vi "main.vi"(8 "error in":errorcluster caption="错误输入") -> (0 "error out":errorcluster caption="错误输出", 3 "task out":refnum<k21> caption="任务输出")   [LabVIEW 2019]
uses:
  <vilib>/DAQmx/create/channels.llb/DAQmx Create Channel (AI-Voltage-Basic).vi
  <vilib>/DAQmx/configure/timing.llb/DAQmx Timing (Sample Clock).vi
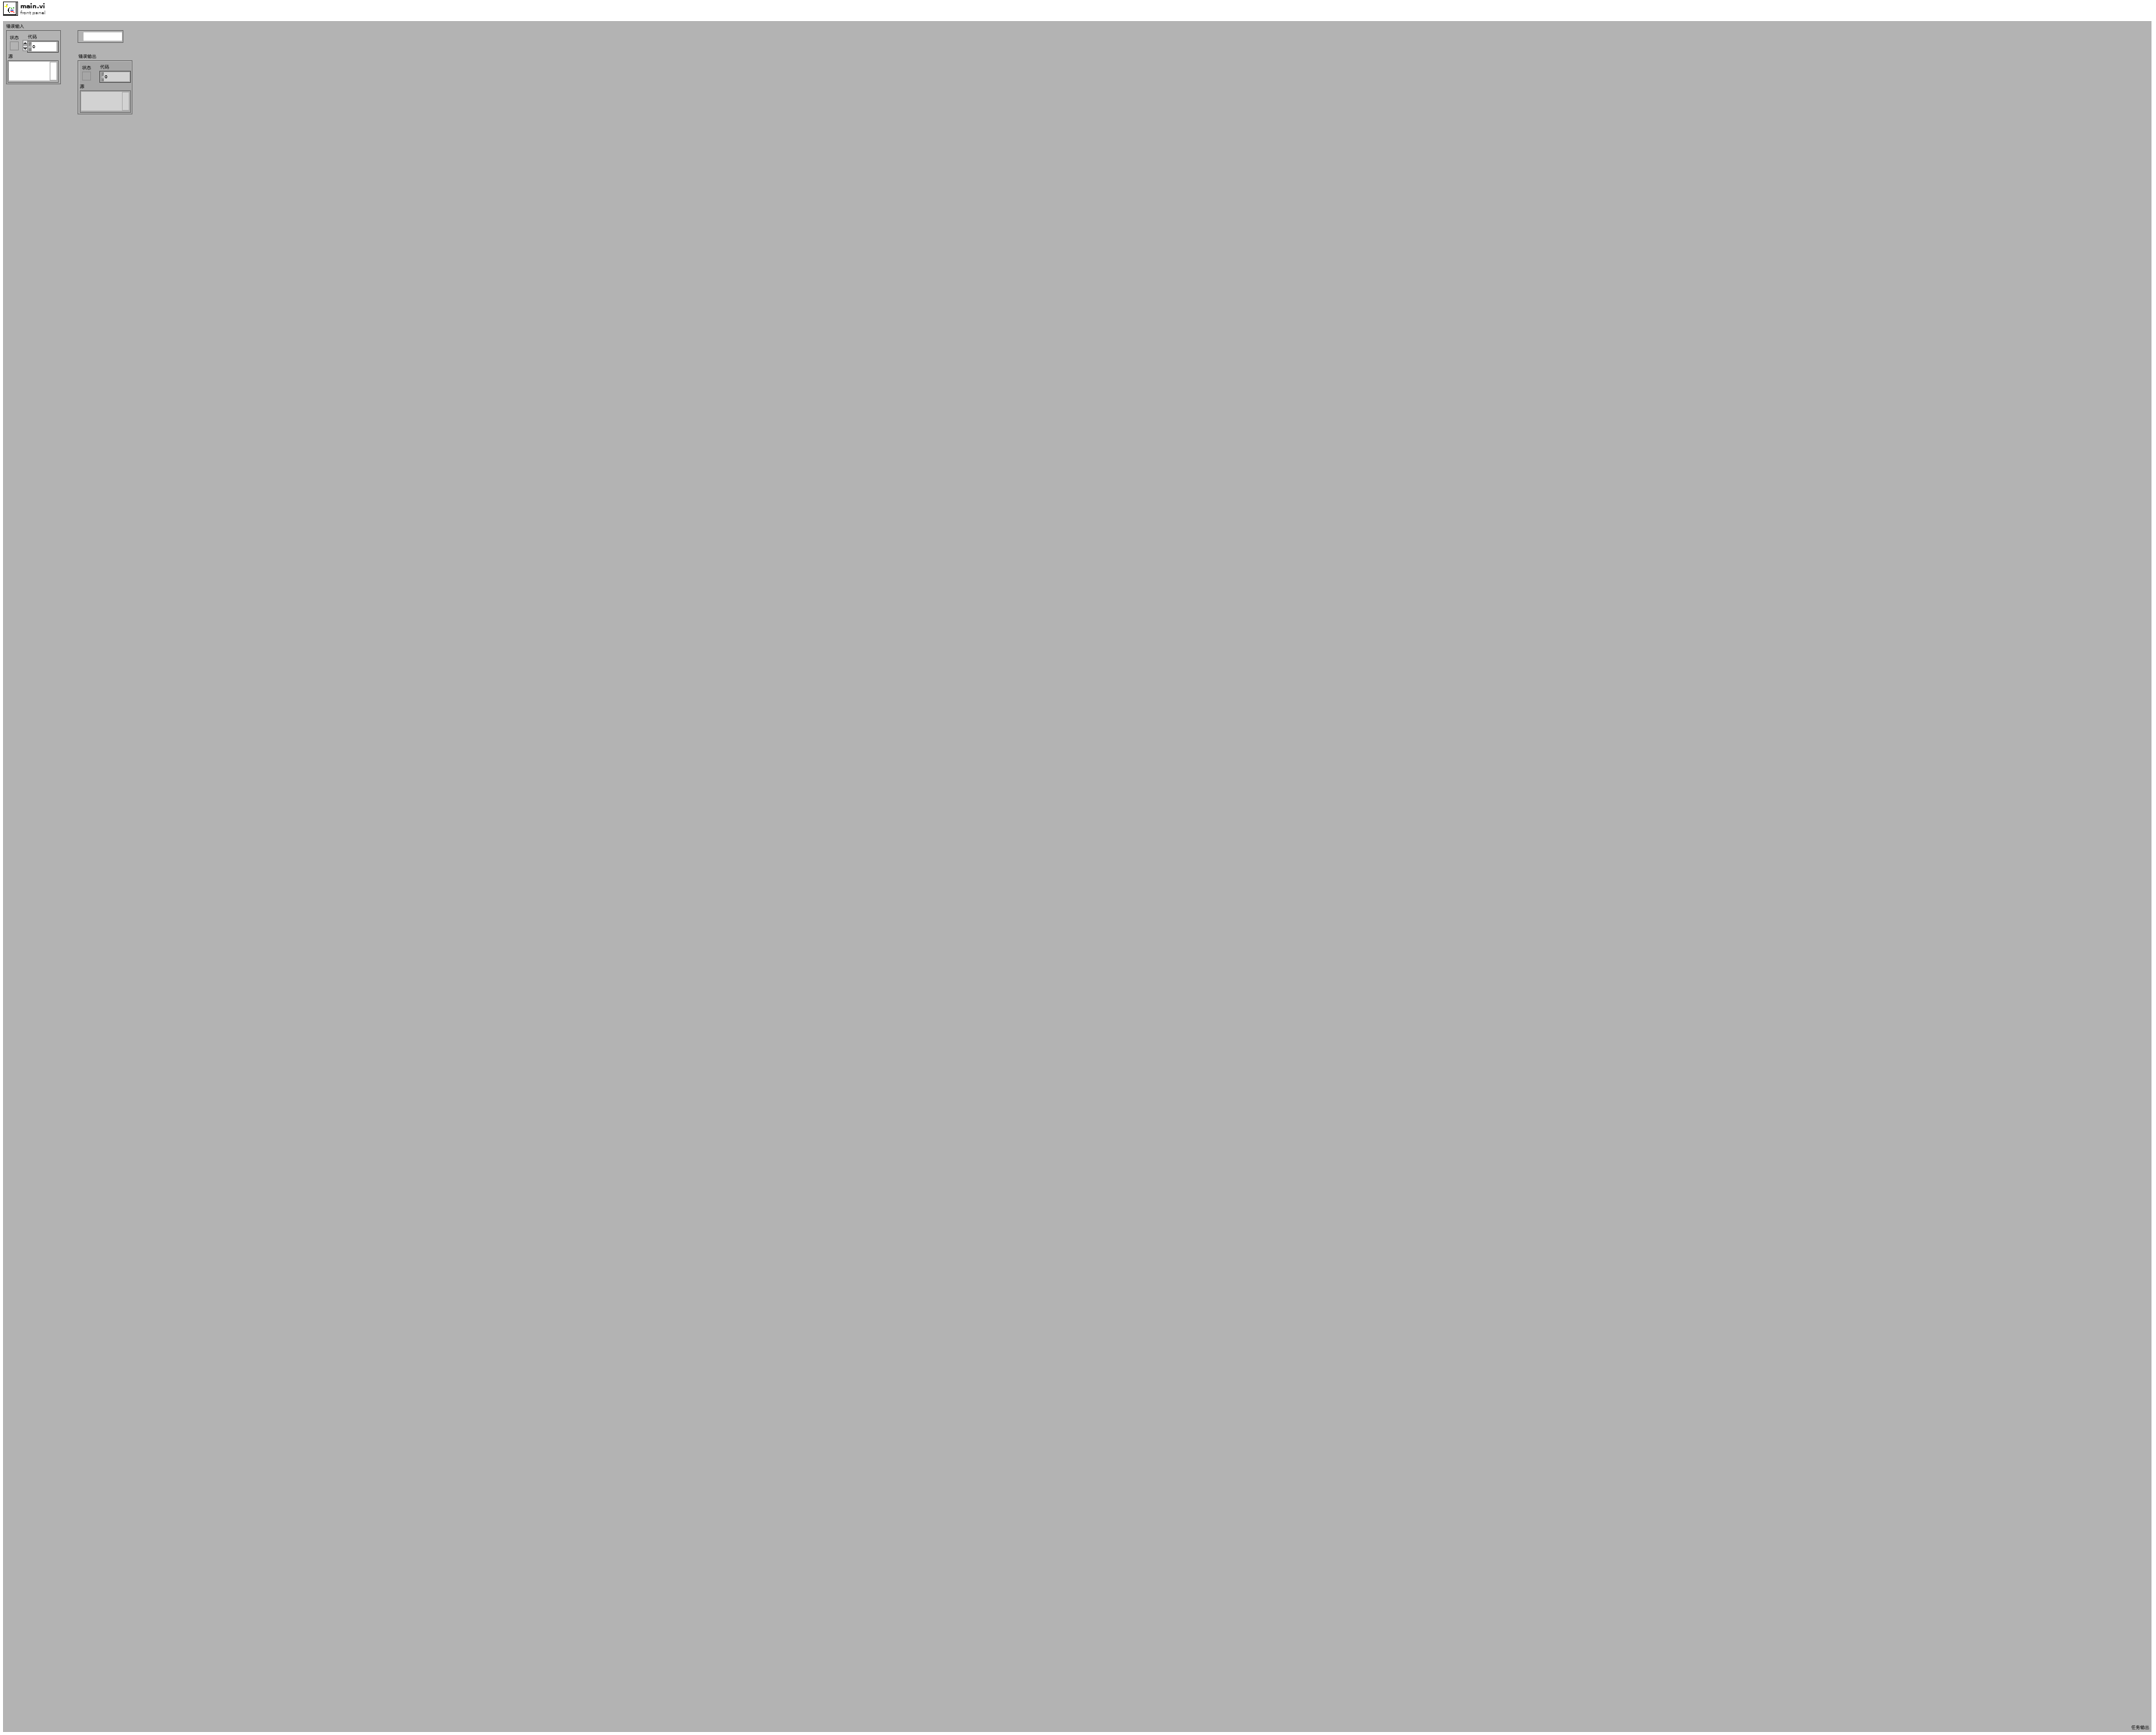
[diagram p1: front panel]
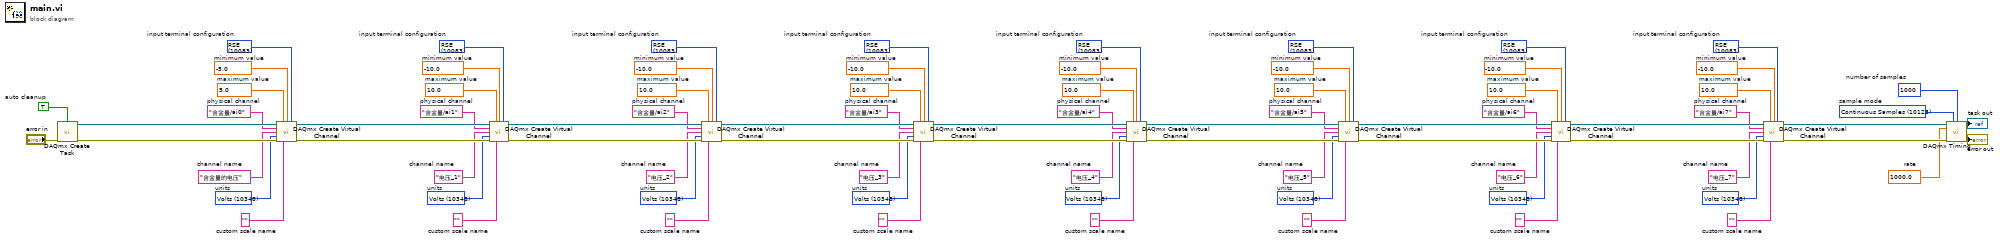
[diagram p0: block diagram]
diagram:
  w1 = 10123 items=["Finite Samples"=10178, "Continuous Samples"=10123, "Hardware Timed Single Point"=12522]  # sample mode
  w2 = 1000  # number of samples
  w3 = 1000.0  # rate
  w7 = 10083 items=["default"=-1, "RSE"=10083, "NRSE"=10078, "Differential"=10106, "Pseudodifferential"=12529]  # input terminal configuration
  w8 = 10348 items=["Volts"=10348, "From Custom Scale"=10065]  # units
  w9 = "电压_7"  # channel name
  w11 = ""  # custom scale name
  w12 = -10.0  # minimum value
  w13 = 10.0  # maximum value
  w14 = "含金量/ai7"  # physical channel
  w16 = 10083 items=["default"=-1, "RSE"=10083, "NRSE"=10078, "Differential"=10106, "Pseudodifferential"=12529]  # input terminal configuration
  w17 = 10348 items=["Volts"=10348, "From Custom Scale"=10065]  # units
  w18 = "电压_6"  # channel name
  w20 = ""  # custom scale name
  w21 = -10.0  # minimum value
  w22 = 10.0  # maximum value
  w23 = "含金量/ai6"  # physical channel
  w25 = 10083 items=["default"=-1, "RSE"=10083, "NRSE"=10078, "Differential"=10106, "Pseudodifferential"=12529]  # input terminal configuration
  w26 = 10348 items=["Volts"=10348, "From Custom Scale"=10065]  # units
  w27 = "电压_5"  # channel name
  w29 = ""  # custom scale name
  w30 = -10.0  # minimum value
  w31 = 10.0  # maximum value
  w32 = "含金量/ai5"  # physical channel
  w34 = 10083 items=["default"=-1, "RSE"=10083, "NRSE"=10078, "Differential"=10106, "Pseudodifferential"=12529]  # input terminal configuration
  w35 = 10348 items=["Volts"=10348, "From Custom Scale"=10065]  # units
  w36 = "电压_4"  # channel name
  w38 = ""  # custom scale name
  w39 = -10.0  # minimum value
  w40 = 10.0  # maximum value
  w41 = "含金量/ai4"  # physical channel
  w43 = 10083 items=["default"=-1, "RSE"=10083, "NRSE"=10078, "Differential"=10106, "Pseudodifferential"=12529]  # input terminal configuration
  w44 = 10348 items=["Volts"=10348, "From Custom Scale"=10065]  # units
  w45 = "电压_3"  # channel name
  w47 = ""  # custom scale name
  w48 = -10.0  # minimum value
  w49 = 10.0  # maximum value
  w50 = "含金量/ai3"  # physical channel
  w52 = 10083 items=["default"=-1, "RSE"=10083, "NRSE"=10078, "Differential"=10106, "Pseudodifferential"=12529]  # input terminal configuration
  w53 = 10348 items=["Volts"=10348, "From Custom Scale"=10065]  # units
  w54 = "电压_2"  # channel name
  w56 = ""  # custom scale name
  w57 = -10.0  # minimum value
  w58 = 10.0  # maximum value
  w59 = "含金量/ai2"  # physical channel
  w61 = 10083 items=["default"=-1, "RSE"=10083, "NRSE"=10078, "Differential"=10106, "Pseudodifferential"=12529]  # input terminal configuration
  w62 = 10348 items=["Volts"=10348, "From Custom Scale"=10065]  # units
  w63 = "电压_1"  # channel name
  w65 = ""  # custom scale name
  w66 = -10.0  # minimum value
  w67 = 10.0  # maximum value
  w68 = "含金量/ai1"  # physical channel
  w70 = 10083 items=["default"=-1, "RSE"=10083, "NRSE"=10078, "Differential"=10106, "Pseudodifferential"=12529]  # input terminal configuration
  w71 = 10348 items=["Volts"=10348, "From Custom Scale"=10065]  # units
  w72 = "含金量的电压"  # channel name
  w74 = ""  # custom scale name
  w75 = -5.0  # minimum value
  w76 = 5.0  # maximum value
  w77 = "含金量/ai0"  # physical channel
  w79 = TRUE  # auto cleanup
  n1 = call <vilib>:"DAQmx Create Task.vi"("auto cleanup"=w79, "error in"="error in") -> ("task out"=w78:refnum<k21>, "error out"=w80:errorcluster)  [unwired: 12 in]
  n2 = call-poly <vilib>:"DAQmx Create Virtual Channel.vi"("task in"=w78, "maximum value"=w76, "minimum value"=w75, "input terminal configuration"=w70, "physical channels"=w77, "name to assign"=w72, "units"=w71, "error in"=w80, "custom scale name"=w74) -> ("task out"=w69:refnum<k21>, "error out"=w73:errorcluster)  [unwired: 5 in]
  n3 = call-poly <vilib>:"DAQmx Create Virtual Channel.vi"("task in"=w69, "maximum value"=w67, "minimum value"=w66, "input terminal configuration"=w61, "physical channels"=w68, "name to assign"=w63, "units"=w62, "error in"=w73, "custom scale name"=w65) -> ("task out"=w60:refnum<k21>, "error out"=w64:errorcluster)  [unwired: 5 in]
  n4 = call-poly <vilib>:"DAQmx Create Virtual Channel.vi"("task in"=w60, "maximum value"=w58, "minimum value"=w57, "input terminal configuration"=w52, "physical channels"=w59, "name to assign"=w54, "units"=w53, "error in"=w64, "custom scale name"=w56) -> ("task out"=w51:refnum<k21>, "error out"=w55:errorcluster)  [unwired: 5 in]
  n5 = call-poly <vilib>:"DAQmx Create Virtual Channel.vi"("task in"=w51, "maximum value"=w49, "minimum value"=w48, "input terminal configuration"=w43, "physical channels"=w50, "name to assign"=w45, "units"=w44, "error in"=w55, "custom scale name"=w47) -> ("task out"=w42:refnum<k21>, "error out"=w46:errorcluster)  [unwired: 5 in]
  n6 = call-poly <vilib>:"DAQmx Create Virtual Channel.vi"("task in"=w42, "maximum value"=w40, "minimum value"=w39, "input terminal configuration"=w34, "physical channels"=w41, "name to assign"=w36, "units"=w35, "error in"=w46, "custom scale name"=w38) -> ("task out"=w33:refnum<k21>, "error out"=w37:errorcluster)  [unwired: 5 in]
  n7 = call-poly <vilib>:"DAQmx Create Virtual Channel.vi"("task in"=w33, "maximum value"=w31, "minimum value"=w30, "input terminal configuration"=w25, "physical channels"=w32, "name to assign"=w27, "units"=w26, "error in"=w37, "custom scale name"=w29) -> ("task out"=w24:refnum<k21>, "error out"=w28:errorcluster)  [unwired: 5 in]
  n8 = call-poly <vilib>:"DAQmx Create Virtual Channel.vi"("task in"=w24, "maximum value"=w22, "minimum value"=w21, "input terminal configuration"=w16, "physical channels"=w23, "name to assign"=w18, "units"=w17, "error in"=w28, "custom scale name"=w20) -> ("task out"=w15:refnum<k21>, "error out"=w19:errorcluster)  [unwired: 5 in]
  n9 = call-poly <vilib>:"DAQmx Create Virtual Channel.vi"("task in"=w15, "maximum value"=w13, "minimum value"=w12, "input terminal configuration"=w7, "physical channels"=w14, "name to assign"=w9, "units"=w8, "error in"=w19, "custom scale name"=w11) -> ("task out"=w4:refnum<k21>, "error out"=w10:errorcluster)  [unwired: 5 in]
  n10 = call-poly <vilib>:"DAQmx Timing.vi"("task/channels in"=w4, "sample mode"=w1, "samples per channel"=w2, "rate"=w3, "error in"=w10) -> ("task out"=→"task out":refnum<k21>, "error out"=→"error out":errorcluster)  [unwired: 9 in]
